vi "ChassisSystemUpdateJoystickState.vi"(3 "Rotation Axis Value":dbl, 4 "Joystick Y Axis Value":dbl, 5 "Joystick X Axis Value":dbl) -> (0 "Rotation Status":u16(ring) items=["no Rotation motor output", "Turn Right", "Turn Left"], 1 "Y Status":u16(ring) items=["no Y motor output", "Drive Forward", "Drive Backward"], 2 "X Status":u16(ring) items=["no X motor output", "Strafe Right", "Strafe Left"])   [LabVIEW 2014]
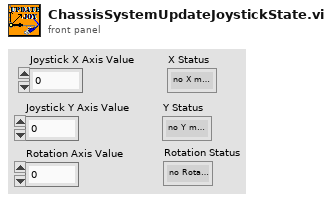
[diagram p1: front panel]
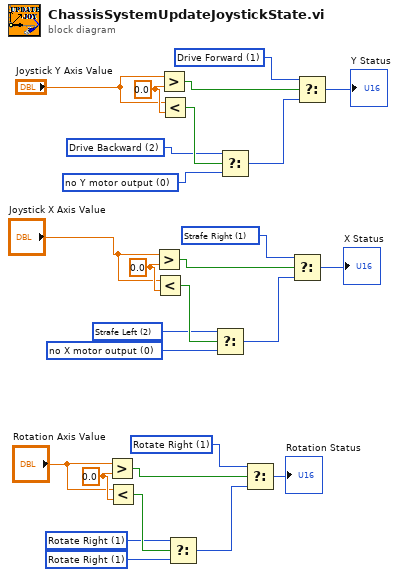
[diagram p0: block diagram]
diagram:
  w2 = u16 1 items=["no Rotation motor output", "Rotate Right", "Rotate Left"] ("Y status")
  w3 = u16 1 items=["no Rotation motor output", "Rotate Right", "Rotate Left"] ("Y status")
  w5 = u16 1 items=["no Rotation motor output", "Rotate Right", "Rotate Left"] ("Y status")
  w8 = 0.0 ("y")
  w11 = u16 0 items=["no X motor output", "Strafe Right", "Strafe Left"] ("Y status")
  w12 = u16 2 items=["no X motor output", "Strafe Right", "Strafe Left"] ("Y status")
  w14 = u16 1 items=["no X motor output", "Strafe Right", "Strafe Left"] ("Y status")
  w17 = 0.0 ("y")
  w20 = u16 1 items=["no Y motor output", "Drive Forward", "Drive Backward"] ("Y status")
  w21 = u16 2 items=["no Y motor output", "Drive Forward", "Drive Backward"] ("Y status")
  w22 = u16 0 items=["no Y motor output", "Drive Forward", "Drive Backward"] ("Y status")
  w26 = 0.0 ("y")
  n1 = Greater?(x="Rotation Axis Value", y=w8) -> (0:w9:bool)
  n2 = Less?(x="Rotation Axis Value", y=w8) -> (x < y?=w7:bool)
  n3 = Greater?(x="Joystick X Axis Value", y=w17) -> (0:w18:bool)
  n4 = Less?(x="Joystick X Axis Value", y=w17) -> (x < y?=w16:bool)
  n5 = Greater?(x="Joystick Y Axis Value", y=w26) -> (0:w27:bool)
  n6 = Less?(x="Joystick Y Axis Value", y=w26) -> (x < y?=w25:bool)
  n7 = Select(t=w3, s=w7, f=w2) -> (s? t:f=w6:u16)
  n8 = Select(t=w12, s=w16, f=w11) -> (s? t:f=w15:u16)
  n9 = Select(t=w21, s=w25, f=w22) -> (s? t:f=w24:u16)
  n10 = Select(t=w5, s=w9, f=w6) -> (s? t:f=→"Rotation Status":u16)
  n11 = Select(t=w14, s=w18, f=w15) -> (s? t:f=→"X Status":u16)
  n12 = Select(t=w20, s=w27, f=w24) -> (s? t:f=→"Y Status":u16)
